vi "getValue.vi"(8 "error in (no error)":errorcluster, 11 "type.U8 in":refnum<class "type.DBL.lvclass">) -> (0 "error out":errorcluster, 2 "value":variant, 3 "type.U8 out":refnum<class "type.DBL.lvclass">)   [LabVIEW 2013, in "type.DBL.lvclass"]
uses:
  type.DBL.lvclass
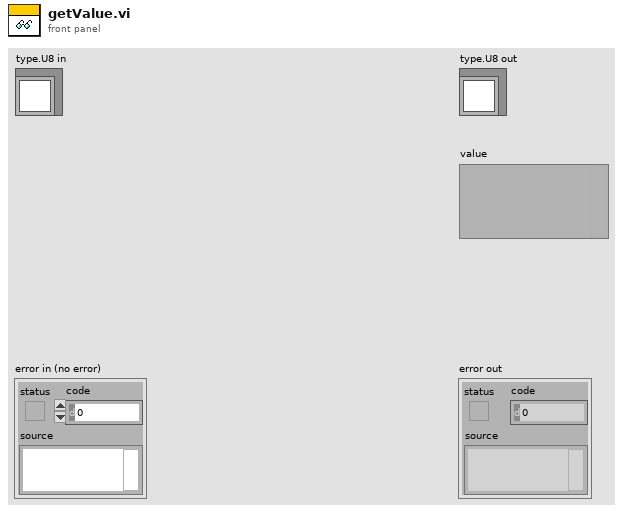
[diagram p1: front panel]
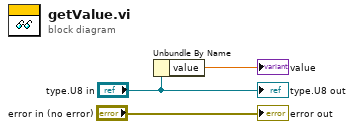
[diagram p0: block diagram]
diagram:
  n1 = Unbundle By Name("type.U8 in") -> ("value"=→"value":dbl)
  "error out" <- "error in (no error)"
  "type.U8 out" <- "type.U8 in"
